vi "OtherJoystick.vi"() -> (3 "Stop":bool)   [LabVIEW 2015]
uses:
  <vilib>/Utility/inputDevices.llb/joystickAcquire.vi
  <vilib>/Utility/inputDevices.llb/closeJoystick.vi
panel:
  in  "stop 3":bool
  in  "stop 2":bool
  out "Other Joystick":T1
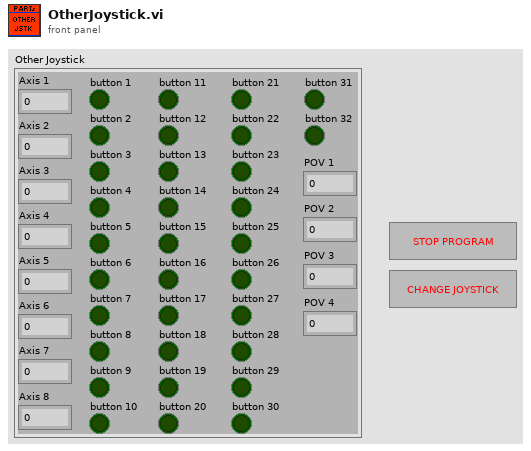
[diagram p1: front panel]
types:
  T1 = cluster{"Axis 1":i32, "Axis 2":i32, "Axis 3":i32, "Axis 4":i32, "Axis 5":i32, "Axis 6":i32, "Axis 7":i32, "Axis 8":i32, "button 1":bool, "button 2":bool, "button 3":bool, "button 4":bool, "button 5":bool, "button 6":bool, "button 7":bool, "button 8":bool, "button 9":bool, "button 10":bool, "button 11":bool, "button 12":bool, "button 13":bool, "button 14":bool, "button 15":bool, "button 16":bool, "button 17":bool, "button 18":bool, "button 19":bool, "button 20":bool, "button 21":bool, "button 22":bool, "button 23":bool, "button 24":bool, "button 25":bool, "button 26":bool, "button 27":bool, "button 28":bool, "button 29":bool, "button 30":bool, "button 31":bool, "button 32":bool, "POV 1":i32, "POV 2":i32, "POV 3":i32, "POV 4":i32}
  T2 = cluster{"X axis":i32, "Y axis":i32, "Z axis":i32, "X axis rotation":i32, "Y axis rotation":i32, "Z axis rotation":i32, "U axis":i32, "V axis":i32}
  T3 = cluster{"button 1":bool, "button 2":bool, "button 3":bool, "button 4":bool, "button 5":bool, "button 6":bool, "button 7":bool, "button 8":bool, "button 9":bool, "button 10":bool, "button 11":bool, "button 12":bool, "button 13":bool, "button 14":bool, "button 15":bool, "button 16":bool, "button 17":bool, "button 18":bool, "button 19":bool, "button 20":bool, "button 21":bool, "button 22":bool, "button 23":bool, "button 24":bool, "button 25":bool, "button 26":bool, "button 27":bool, "button 28":bool, "button 29":bool, "button 30":bool, "button 31":bool, "button 32":bool}
  T4 = cluster{"pov 1":i32, "pov 2":i32, "pov 3":i32, "pov 4":i32}
  T5 = cluster{"X axis":i32, "Y axis":i32, "Z axis":i32, "X axis rotation":i32, "Y axis rotation":i32, "Z axis rotation":i32, "U axis":i32, "V axis":i32, "button 1":bool, "button 2":bool, "button 3":bool, "button 4":bool, "button 5":bool, "button 6":bool, "button 7":bool, "button 8":bool, "button 9":bool, "button 10":bool, "button 11":bool, "button 12":bool, "button 13":bool, "button 14":bool, "button 15":bool, "button 16":bool, "button 17":bool, "button 18":bool, "button 19":bool, "button 20":bool, "button 21":bool, "button 22":bool, "button 23":bool, "button 24":bool, "button 25":bool, "button 26":bool, "button 27":bool, "button 28":bool, "button 29":bool, "button 30":bool, "button 31":bool, "button 32":bool, "pov 1":i32, "pov 2":i32, "pov 3":i32, "pov 4":i32}
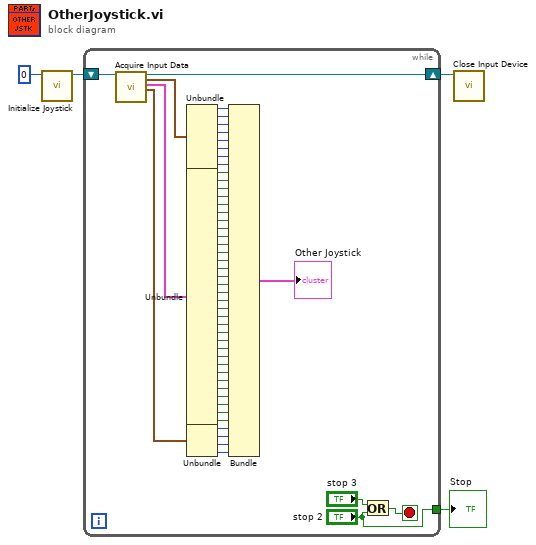
[diagram p0: block diagram]
diagram:
  n1 = call <vilib>:"Initialize Joystick.vi"("device index"=0) -> ("device ID"=w4:refnum<k1>)  [unwired: 9 in, 1 out]
  n2 = while {
    shift-right: [w56] -> w2
    shift-left: w4 -> [w57]
    tunnel: ["stop 2"] -> w1
    stop <- w6 stop-if-true
    n3 = call-poly <vilib>:"Acquire Input Data.vi"("device ID"=w57) -> ("device ID"=w56:refnum<k1>, "axis info"=w55:T2, "button info"=w54:T3, "direction info"=w53:T4)  [unwired: 14 in, 1 out]
    n4 = Unbundle(w55) -> ("X axis"=w52:i32, "Y axis"=w51:i32, "Z axis"=w50:i32, "X axis rotation"=w49:i32, "Y axis rotation"=w48:i32, "Z axis rotation"=w47:i32, "U axis"=w46:i32, "V axis"=w45:i32)
    n5 = Unbundle(w54) -> ("button 1"=w44:bool, "button 2"=w43:bool, "button 3"=w42:bool, "button 4"=w41:bool, "button 5"=w40:bool, "button 6"=w39:bool, "button 7"=w38:bool, "button 8"=w37:bool, "button 9"=w36:bool, "button 10"=w35:bool, "button 11"=w34:bool, "button 12"=w33:bool, "button 13"=w32:bool, "button 14"=w31:bool, "button 15"=w30:bool, "button 16"=w29:bool, "button 17"=w28:bool, "button 18"=w27:bool, "button 19"=w26:bool, "button 20"=w25:bool, "button 21"=w24:bool, "button 22"=w23:bool, "button 23"=w22:bool, "button 24"=w21:bool, "button 25"=w20:bool, "button 26"=w19:bool, "button 27"=w18:bool, "button 28"=w17:bool, "button 29"=w16:bool, "button 30"=w15:bool, "button 31"=w14:bool, "button 32"=w13:bool)
    n6 = Unbundle(w53) -> ("pov 1"=w12:i32, "pov 2"=w11:i32, "pov 3"=w10:i32, "pov 4"=w9:i32)
    n7 = Bundle("X axis"=w52, "Y axis"=w51, "Z axis"=w50, "X axis rotation"=w49, "Y axis rotation"=w48, "Z axis rotation"=w47, "U axis"=w46, "V axis"=w45, "button 1"=w44, "button 2"=w43, "button 3"=w42, "button 4"=w41, "button 5"=w40, "button 6"=w39, "button 7"=w38, "button 8"=w37, "button 9"=w36, "button 10"=w35, "button 11"=w34, "button 12"=w33, "button 13"=w32, "button 14"=w31, "button 15"=w30, "button 16"=w29, "button 17"=w28, "button 18"=w27, "button 19"=w26, "button 20"=w25, "button 21"=w24, "button 22"=w23, "button 23"=w22, "button 24"=w21, "button 25"=w20, "button 26"=w19, "button 27"=w18, "button 28"=w17, "button 29"=w16, "button 30"=w15, "button 31"=w14, "button 32"=w13, "pov 1"=w12, "pov 2"=w11, "pov 3"=w10, "pov 4"=w9) -> (→"Other Joystick":T5)  [unwired: 1 in]
    n8 = Or(x="stop 3", y="stop 2") -> (x .or. y?=w6:bool)
  }
  "Stop" <- w1
  n9 = call-poly <vilib>:"Close Input Device.vi"("device ID"=w2) -> ()  [unwired: 9 in, 1 out]
